vi "remote.Commit Properties (Generic).vi"(0 "SLSC Remote in":refnum<class "SLSC Remote.lvclass">, 5 "resources":string, 11 "error in (no error)":errorcluster) -> (4 "SLSC Remote out":refnum<class "SLSC Remote.lvclass">, 15 "error out":errorcluster)   [LabVIEW 2016, in "SLSC Interfaces.lvlib" / "SLSC Remote.lvclass"]
uses:
  SLSC Remote.lvclass
  <vilib>/NI/NI JSONRPC Server Framework/Classes/Server/JSONRPC Server.lvclass
  <vilib>/httpClient/LabVIEWHTTPClient.lvlib
  <vilib>/httpClient/POSTBuffer.vi
  <vilib>/NI/JSON Support for LabVIEW/JSON Data Classes/JSON Helper/JSON Helper.lvclass
  <vilib>/NI/JSON Support for LabVIEW/JSON Data Classes/JSON Object/JSON Object.lvclass
  <vilib>/NI/JSON Support for LabVIEW/JSON Data Classes/JSON Object/Insert Key Value Pair (Single String).vi
  <vilib>/NI/JSON Support for LabVIEW/JSON Data Classes/JSON Object/New JSON Object (Empty).vi
  <vilib>/NI/NI JSONRPC Server Framework/Classes/Server/Format Client Request (Auto-Increment).vi
  <vilib>/NI/NI JSONRPC Server Framework/Classes/Server/Parse Response (Object).vi
  C:/Program Files (x86)/National Instruments/LabVIEW 2016/vi.lib/NI/JSON Support for LabVIEW/JSON Data Classes/JSON Structured Type/JSON Structure.lvclass
  C:/Program Files (x86)/National Instruments/LabVIEW 2016/vi.lib/NI/JSON Support for LabVIEW/JSON Data Classes/JSON Datatype/JSON Null.lvclass
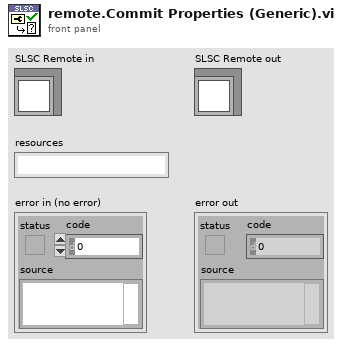
[diagram p1: front panel]
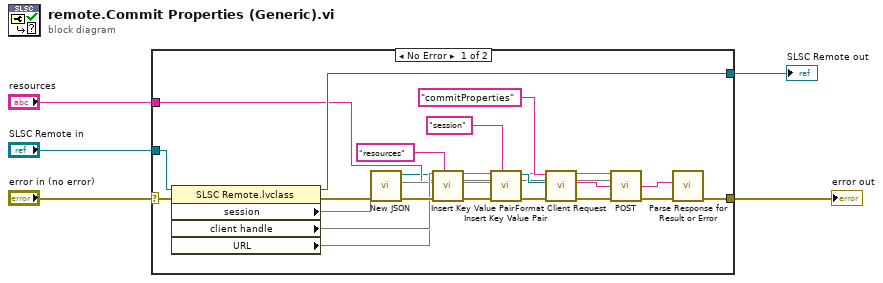
[diagram p0: block diagram]
diagram:
  n1 = case shown="No Error" "error in (no error)" {
    selector: "error in (no error)" -> [w25 w28]
    tunnel: "resources" -> [w8 _]
    tunnel: "SLSC Remote in" -> [w27 w29]
    tunnel: [w26 w29] -> w2
    tunnel: [w12 w28] -> w1
    frame No Error {
      n2 = property class="SLSC Remote.lvclass"(reference=w27, error in=w25) -> (reference out=w26:refnum<class "SLSC Remote.lvclass">, error out=w24:errorcluster, "session"=w11, "client handle"=w17, "URL"=w16)
      n3 = call-poly <vilib>:"New JSON.vi"("error in (no error)"=w24) -> ("error out"=w23:errorcluster, "JSON Object out"=w7:refnum<class "JSON Object.lvclass">)  [unwired: 9 in]
      n4 = call-poly <vilib>:"Insert Key Value Pair.vi"("key"="resources" ("Name"), "error in (no error)"=w23, "value"=w8, "JSON Object in"=w7) -> ("error out"=w22:errorcluster, "JSON Object out"=w6:refnum<class "JSON Object.lvclass">)  [unwired: 5 in, 1 out]
      n5 = call-poly <vilib>:"Insert Key Value Pair.vi"("key"="session" ("Name"), "error in (no error)"=w22, "value"=w11, "JSON Object in"=w6) -> ("error out"=w18:errorcluster, "JSON Object out"=w19:refnum<class "JSON Object.lvclass">)  [unwired: 5 in, 1 out]
      n6 = call-poly <vilib>:"Format Client Request.vi"("error in (no error)"=w18, "JSON in"=w19, "method"="commitProperties") -> ("error out"=w15:errorcluster, "Request String"=w20:string)  [unwired: 7 in]
      n7 = call-poly <vilib>:"POST.vi"("client handle"=w17, "url"=w16, "buffer"=w20, "error in (no error)"=w15) -> ("body"=w14:string, "error out"=w13:errorcluster)  [unwired: 8 in, 2 out]
      n8 = call-poly <vilib>:"Parse Response for Result or Error.vi"("error in"=w13, "Response String In"=w14) -> ("error out"=w12:errorcluster)  [unwired: 7 in, 2 out]
    }
    frame Error {
    }
  }
  "error out" <- w1
  "SLSC Remote out" <- w2
